vi "Formic Queen.vi"(8 "error in (no error)":errorcluster, 9 "SelfID":i32, 10 "Map":i32[](array[numeric]), 11 "Mother in":refnum<class "Formics.lvclass">) -> (0 "error out":errorcluster, 1 "Direction":T1, 2 "Action":T2, 3 "Mother out":refnum<class "Formics.lvclass">, 4 "Replicated Class":refnum<class "Formics.lvclass">)   [LabVIEW 2015, in "Formics.lvclass"]
uses:
  Formics.lvclass
  Type Defs/Action Enum.ctl
  Type Defs/Direction Enum.ctl
  Formics.lvclass/Formics.ctl
  SquareStatus.ctl
  Formic Types.ctl
  Queen Bee Steps.ctl
  Square/Square.lvclass
panel:
  in  "Protectors":i32[](array[numeric])=[2, 6]
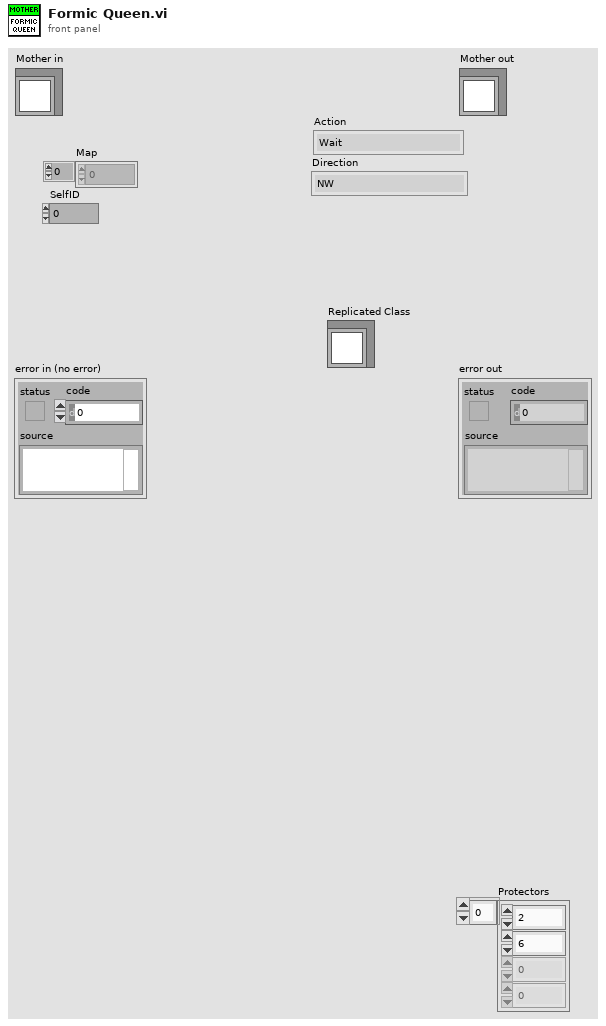
[diagram p1: front panel]
types:
  T1 = typedef "Square.lvclass/Direction Enum.ctl" = enum16{"NW", "N", "NE", "E", "SE", "S", "SW", "W"}
  T2 = typedef "Square.lvclass/Action Enum.ctl" = enum16{"Wait", "Move", "Attack", "Replicate"}
  T3 = typedef "Formics.lvclass/Formic Types.ctl" = enum16{"Queen Bee", "Protector Bee", "Daughter Bee", "Worker Bee", "Coward"}
  T4 = typedef "Formics.lvclass/SquareStatus.ctl" = cluster{"ID":i32, "Heartbeat":bool}
  T5 = typedef "Formics.lvclass/Queen Bee Steps.ctl" = enum16{"Attack?", "Migrate?", "Kamikaze?", "Protect?", "Procreate?", "Build Army"}
  T6 = typedef "Formics.lvclass/Kamikaze DVR.ctl" = refnum<data-value>
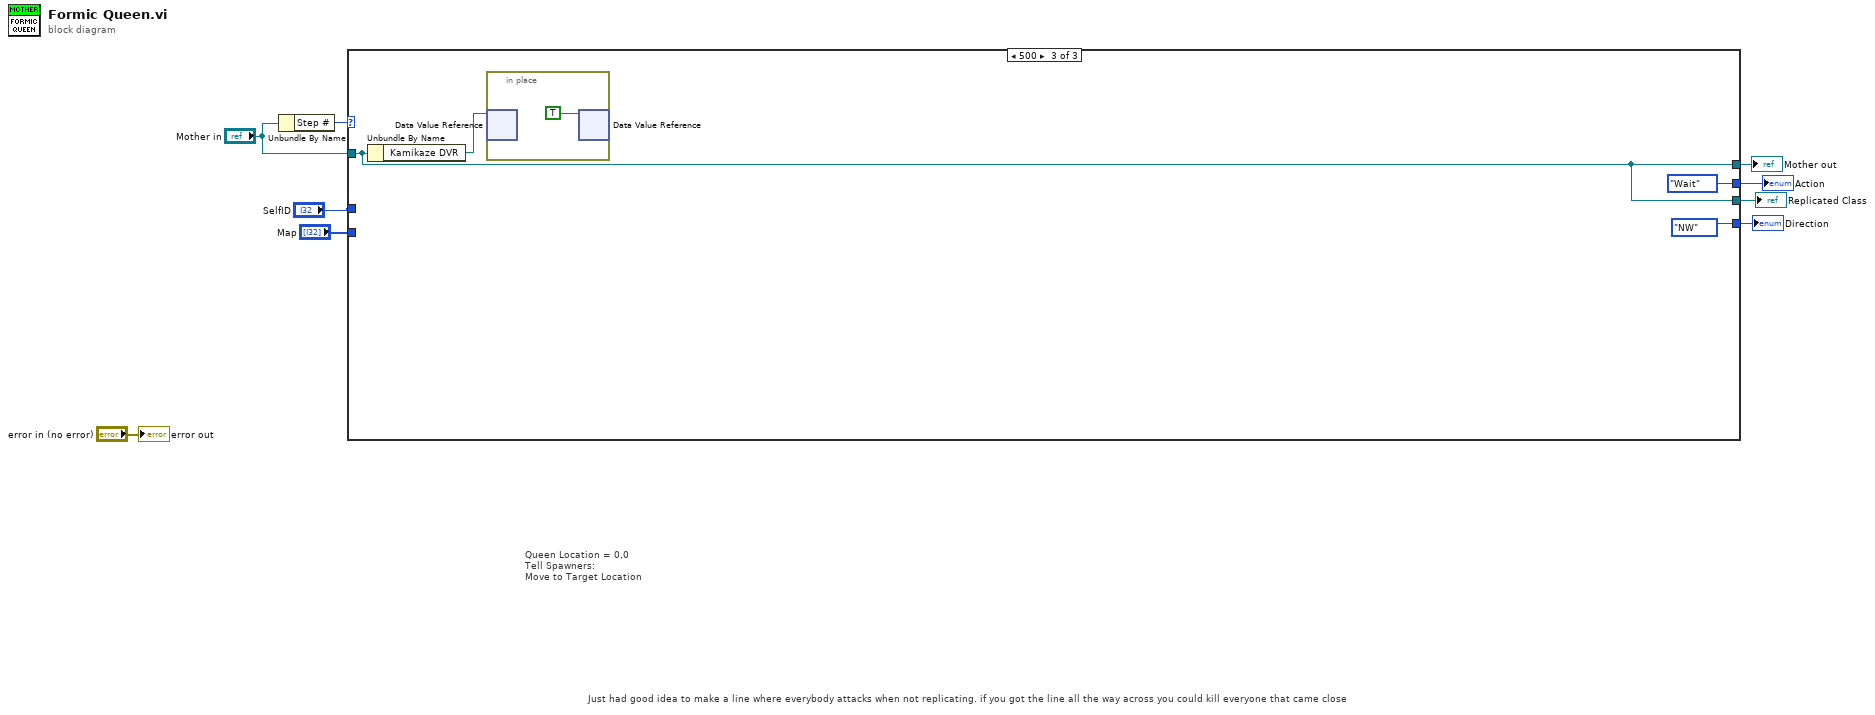
[diagram p0: block diagram]
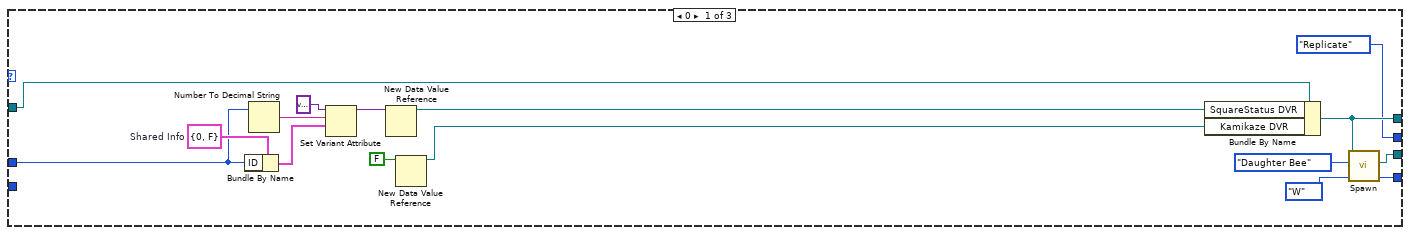
[diagram p2: hidden frame]
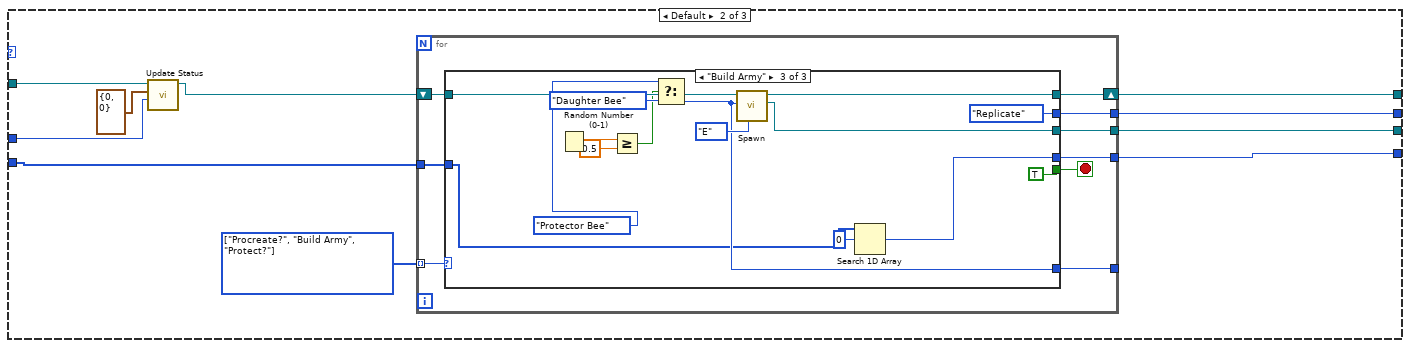
[diagram p3: hidden frame]
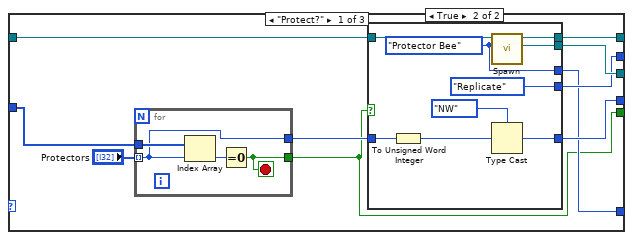
[diagram p4: hidden frame]
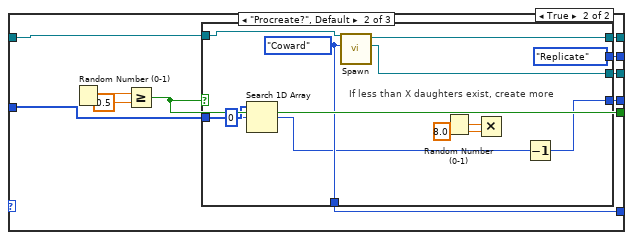
[diagram p6: hidden frame]
diagram:
  # "Just had good idea to make a line where everybody attacks when not replicating. if you got the line all the way across you could kill everyone that came close"
  # "Queen Location = 0,0\nTell Spawners:\nMove to Target Location"
  n1 = Unbundle By Name("Mother in") -> ("Step #"=w6:i32)
  n2 = case shown="500" w6 {
    tunnel: [w14 w30 w106] -> w8
    tunnel: "Mother in" -> [w16 w33 w106]
    tunnel: "SelfID" -> [w15 w32 _]
    tunnel: "Map" -> [_ w28 _]
    tunnel: [Action_Enum."Replicate" ("Action") w27 Action_Enum."Wait" ("Action")] -> w3
    tunnel: [Direction_Enum."W" ("Direction") w26 Direction_Enum."NW" ("Direction")] -> w2
    tunnel: [w11 w25 w106] -> w1
    frame 0 {
      w21 = T4 {"ID"=0, "Heartbeat"=FALSE}  # Shared Info
      n3 = Bundle By Name(cluster=w21, "ID"=w15) -> (w22:T4)
      n4 = Number To Decimal String(number=w15) -> (decimal integer string=w23:string)  [unwired: 1 in]
      n5 = Set Variant Attribute(Variant=variant ("variant"), name=w23, value=w22) -> (Variant out=w20:variant)  [unwired: 1 in, 2 out]
      n6 = New Data Value Reference(data value=w20) -> (data value reference=w19:refnum<data-value>)  [unwired: 1 in, 1 out]
      n7 = New Data Value Reference(data value=FALSE) -> (data value reference=w18:refnum<data-value>)  [unwired: 1 in, 1 out]
      n8 = Bundle By Name(cluster=w16, "SquareStatus DVR"=w19, "Kamikaze DVR"=w18) -> (w14:refnum<class "Formics.lvclass">)
      n9 = call "Spawn.vi"(10:Formic_Types."Daughter Bee", "Mother in"=w14) -> ("Replicated Class"=w11:refnum<class "Formics.lvclass">)  [unwired: 7 in, 2 out]
    }
    frame Default {
      w29 = T5[] [enum."Procreate?", enum."Build Army", enum."Protect?"] items=["Attack?", "Migrate?", "Kamikaze?", "Protect?", "Procreate?", "Build Army"]
      n10 = call "Update Status.vi"("ID"=w32, "MyPosition"=cluster{"X":i32, "Y":i32} {"X"=0, "Y"=0}, "Mother in"=w33) -> ("Mother out"=w31:refnum<class "Formics.lvclass">)  [unwired: 8 in]
      n11 = for {
        shift-right: [w42] -> w30
        shift-left: w31 -> [w43]
        tunnel: [w41] -> w27
        tunnel: [w40] -> w26
        tunnel: w29 -> [w39] mode=indexing
        tunnel: [w37] -> w25
        tunnel: [w36] -> _
        tunnel: w28 -> [w35]
        stop <- w38 stop-if-true
        n12 = case shown="\"Build Army\"" w39 {
          tunnel: w43 -> [w53 w72 w104]
          tunnel: [w52 w75 w102] -> w42
          tunnel: [w50 w77 Action_Enum."Replicate" ("Action")] -> w41
          tunnel: [w47 w76 w90] -> w40
          tunnel: [w45 w68 TRUE ("Enemy Found?")] -> w38
          tunnel: [w51 w74 w101] -> w37
          tunnel: [w46 w73 w95] -> w36
          tunnel: w35 -> [w44 w69 w92]
          frame "Protect?" {
            n13 = for {
              tunnel: w44 -> [w67]
              tunnel: [w66] -> w45
              tunnel: "Protectors" -> [w64] mode=indexing
              tunnel: [w64] -> w48
              stop <- w66 stop-if-true
              n14 = Index Array(array=w67, index=w64) -> (element=w65:i32)
              n15 = Equal To 0?(x=w65) -> (x = 0?=w66:bool)
            }
            n16 = case shown="True" w45 {
              tunnel: w53 -> [w54 w63]
              tunnel: [w54 w62] -> w52
              tunnel: [_ w61] -> w51
              tunnel: [_ Action_Enum."Replicate" ("Action")] -> w50
              tunnel: w48 -> [_ w58]
              tunnel: [_ w57] -> w47
              tunnel: [_ w55] -> w46
              frame False {
              }
              frame True {
                w55 = Formic_Types."Protector Bee"
                n17 = To Unsigned Word Integer(number=w58) -> (unsigned 16bit integer=w59:u16)
                n18 = call "Spawn.vi"(10:w55, "Mother in"=w63) -> ("Replicated Class"=w61:refnum<class "Formics.lvclass">, "Mother out"=w62:refnum<class "Formics.lvclass">)  [unwired: 7 in, 1 out]
                n19 = Type Cast(type=Direction_Enum."NW" ("Direction"), x=w59) -> (*(type *) &x=w57:T1)
              }
            }
          }
          frame "Procreate?", Default {
            n20 = Random Number (0-1)() -> (number: 0 to 1=w71:dbl)
            n21 = Greater Or Equal?(x=w71, y=0.5) -> (x >= y?=w68:bool)
            n22 = case shown="True" w68 {
              tunnel: [_ Action_Enum."Replicate" ("Action")] -> w77
              tunnel: [_ w83] -> w76
              tunnel: [w78 w88] -> w75
              tunnel: [_ w87] -> w74
              tunnel: [_ w86] -> w73
              tunnel: w72 -> [w78 w82]
              tunnel: w69 -> [_ w81]
              frame False {
              }
              frame True {
                w86 = Formic_Types."Coward"
                # "If less than X daughters exist, create more"
                n23 = Search 1D Array(1D array=w81, element=0) -> (index of element=w79:i32)  [unwired: 1 in]
                n24 = call "Spawn.vi"(10:w86, "Mother in"=w82) -> ("Replicated Class"=w87:refnum<class "Formics.lvclass">, "Mother out"=w88:refnum<class "Formics.lvclass">)  [unwired: 7 in, 1 out]
                n25 = Random Number (0-1)() -> (number: 0 to 1=w85:dbl)
                n26 = Multiply(x=w85, y=8.0) -> ()  [unwired: 1 out]
                n27 = Decrement(x=w79) -> (x-1=w83:i32)
              }
            }
          }
          frame "Build Army" {
            n28 = Random Number (0-1)() -> (number: 0 to 1=w96:dbl)
            n29 = Greater Or Equal?(x=w96, y=0.5) -> (x >= y?=w93:bool)
            n30 = Select(t=Formic_Types."Protector Bee", s=w93, f=Formic_Types."Daughter Bee") -> (s? t:f=w95:T3)
            n31 = call "Spawn.vi"("Start Direction"=Direction_Enum."E", 10:w95, "Mother in"=w104) -> ("Replicated Class"=w101:refnum<class "Formics.lvclass">, "Mother out"=w102:refnum<class "Formics.lvclass">)  [unwired: 6 in, 1 out]
            n32 = Search 1D Array(1D array=w92, element=0) -> (index of element=w90:i32)  [unwired: 1 in]
          }
        }
      }
    }
    frame 500 {
      n33 = Unbundle By Name(w106) -> ("Kamikaze DVR"=w108:T6)
      n34 = in-place {
        n35 = in-place-dvr #1(w108) -> ()  [unwired: 2 out]
        n36 = in-place-dvr #1(TRUE ("data value")) -> ()  [unwired: 2 out]
      }
    }
  }
  "Mother out" <- w8
  "Action" <- w3
  "Direction" <- w2
  "Replicated Class" <- w1
  "error out" <- "error in (no error)"
